vi "Cancel Notifications.vi"(8 "error in (no error)":errorcluster, 10 "Clean All?":bool, 11 "Client - Data In":T1) -> (0 "error out":errorcluster, 3 "Client- Data Out":T1)   [LabVIEW 2024]
doc: "Cancels the alarm and event notifications and value change notifications for the client."
uses:
  Controls/Client/Client - Data.ctl
  Shared/Message Queue/Client Message Queues.ctl
  Shared/Message Queue/Message Cluster.ctl
  <vilib>/lvdsc/NI_DSC.lvlib
  Shared/Message Queue.lvlib
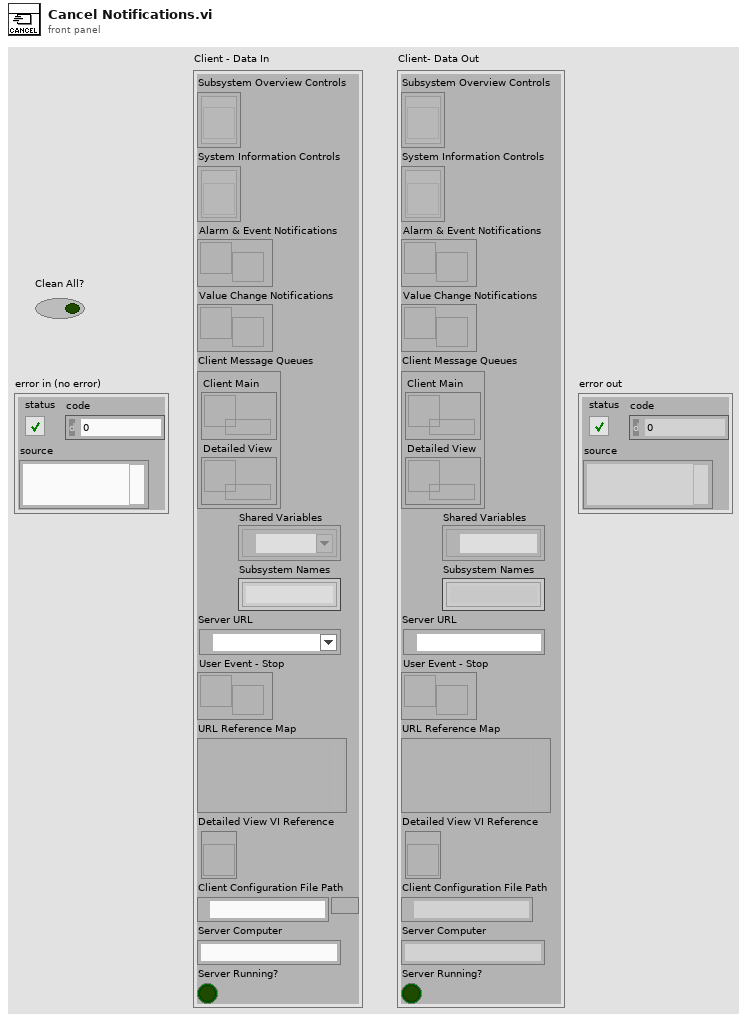
[diagram p1: front panel]
types:
  T1 = typedef "Client - Data.ctl" = cluster{"Subsystem Overview Controls":refnum<vi>[], "System Information Controls":refnum<vi>[], "Alarm & Event Notifications":refnum<user-event>, "Value Change Notifications":refnum<user-event>, "Client Message Queues":T2, "Shared Variables":refnum<k21>[], "Subsystem Names":string[], "Server URL":refnum<k21>, "User Event - Stop":refnum<user-event>, "URL Reference Map":variant, "Detailed View VI Reference":refnum<vi>, "Client Configuration File Path":path, "Server Computer":string, "Server Running?":bool}
  T2 = typedef "Message Queue.lvlib/Client Message Queues.ctl" = cluster{"Client Main":refnum<queue>, "Detailed View":refnum<queue>}
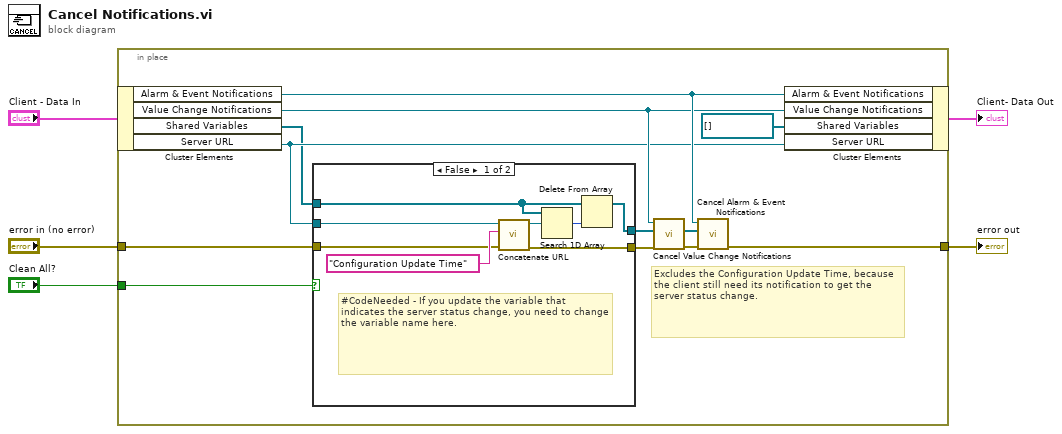
[diagram p0: block diagram]
diagram:
  n1 = in-place {
    in-place-border: "error in (no error)" -> [w11]
    in-place-border: [w12] -> w2
    in-place-border: "Clean All?" -> [w6]
    # "Excludes the Configuration Update Time, because the client still need its notification to get the server status change."
    n2 = in-place-cluster #1("Client - Data In") -> ("Alarm & Event Notifications"=w15:refnum<user-event>, "Value Change Notifications"=w14:refnum<user-event>, "Shared Variables"=w9:refnum<k21>[], "Server URL"=w10:refnum<k21>)
    n3 = case shown="False" w6 {
      tunnel: w11 -> [w24 w26]
      tunnel: w10 -> [w22 _]
      tunnel: w9 -> [w20 w27]
      tunnel: [w19 w27] -> w8
      tunnel: [w18 w26] -> w7
      frame False {
        # "#CodeNeeded - If you update the variable that indicates the server status change, you need to change the variable name here."
        n4 = call "Concatenate URL.vi"("error in (no error)"=w24, "Child Name"="Configuration Update Time", "Parent URL"=w22) -> ("error out"=w18:errorcluster, "Child URL"=w23:refnum<k21>)  [unwired: 7 in]
        n5 = Search 1D Array(1D array=w20, element=w23) -> (index of element=w21:i32)  [unwired: 1 in]
        n6 = Delete From Array(array=w20, index=w21) -> (array with subset deleted=w19:refnum<k21>[])  [unwired: 1 in, 1 out]
      }
      frame True {
      }
    }
    n7 = call <vilib>:"Cancel Value Change Notifications.vi"("error in (no error)"=w7, "shared variables"=w8, "notification refnum"=w14) -> ("error out"=w16:errorcluster, "shared variables out"=w17:refnum<k21>[])  [unwired: 6 in, 1 out]
    n8 = call <vilib>:"Cancel Alarm & Event Notifications.vi"("error in (no error)"=w16, "shared variables"=w17, "notification refnum"=w15) -> ("error out"=w12:errorcluster)  [unwired: 6 in, 2 out]
    n9 = in-place-cluster #1("Alarm & Event Notifications"=w15, "Value Change Notifications"=w14, "Shared Variables"=refnum<k21>[] [] ("shared variables"), "Server URL"=w10) -> (→"Client- Data Out":T1)
  }
  "error out" <- w2
